vi "AlGaInPAs_prep_run_cont_dil_v11.vi"(2 "Debug Mode":bool, 3 "Elapsed Time(s)":dbl, 4 "State":enum16{"Edit", "Start", "Run", "End", "Idle"}(ring), 5 "Argument List In":string[](array[string])) -> (0 "Status Out":string, 1 "Argument List Out":string[](array[string]))   [LabVIEW 2011]
panel:
  out "GAMFC1 set val":dbl caption="R1 (0-10 sscm)" format="%.2f"
  out "Prep-In var":bool
  out "Prep-Ga var":bool
  out "Prep-Al var":bool
  out "Prep-P var":bool
  out "Prep-As var":bool
  out "prep_done":bool
  out "run started":bool
  out "first":bool=TRUE
  out "total time":dbl
  out "is OK?":bool
  out "AsH3?":bool
  out "PH3?":bool
  out "In?":bool
  out "Ga?":bool
  out "Al?":bool
  in  "Prep As":bool caption="Pre-run"
  in  "Prep P":bool caption="Pre-run"
  in  "Prep In":bool caption="Pre-run"
  in  "prep_time":dbl caption="pre-run time (s)"
  in  "Prep Al":bool caption="Pre-run"
  in  "Run As":bool caption="Run"
  in  "AsH3 Flow":dbl caption="AsH3 Flow (0-10 sccm)" format="%.2f"
  in  "P Flow":dbl caption="P Flow (0-100 sccm)" format="%.2f"
  in  "Run P":bool caption="Run"
  in  "In Flow":dbl caption="In Flow (0-100 sscm)" format="%.2f"
  in  "Run In":bool caption="Run"
  in  "Run Al":bool caption="Run"
  in  "Al Flow":dbl caption="Al Flow (0-100 sscm)" format="%.2f"
  in  "Cancel":bool
  in  "OK":bool
  out "tTotal(s) 2":dbl
  in  "Ga Tab Control":enum32{"Page 1", "Page 2"}(tab)
  in  "Ga Dilution":bool caption="Dilute"
  in  "Ga Flow":dbl caption="Ga Flow (0-10 sscm)" format="%.2f"
  in  "Run Ga":bool caption="Run"
  in  "Prep Ga":bool caption="Pre-run"
  in  "GAMFC1":dbl=1.0 caption="R1 (0-10 sscm)" format="%.2f"
  out "GAMFC2 set":dbl caption="R2 (0-100 sscm)" format="%.2f"
  in  "GAMFC3":dbl=100.0 caption="R3 (0-1000 sscm)" format="%.1f"
  out "GAMFC1 set":dbl caption="R1 (0-10 sscm)" format="%.2f"
  # "Add pre-run time to run time in editor."
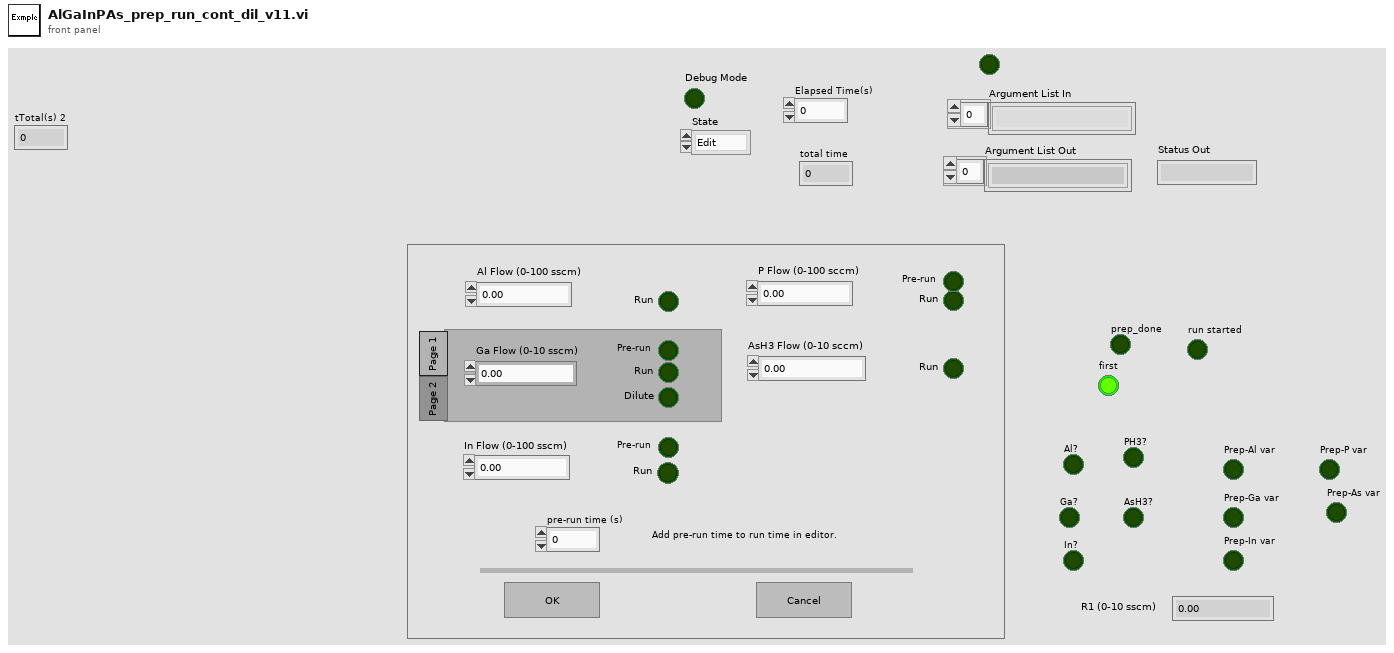
[diagram p1: front panel]
types:
  T1 = enum16{"Discrete", "Continuous", "Instantaneous", "Finite"}
  T2 = enum32{"Invalid", "Default", "Floating", "Floating/Auto-Hide", "Modal"}
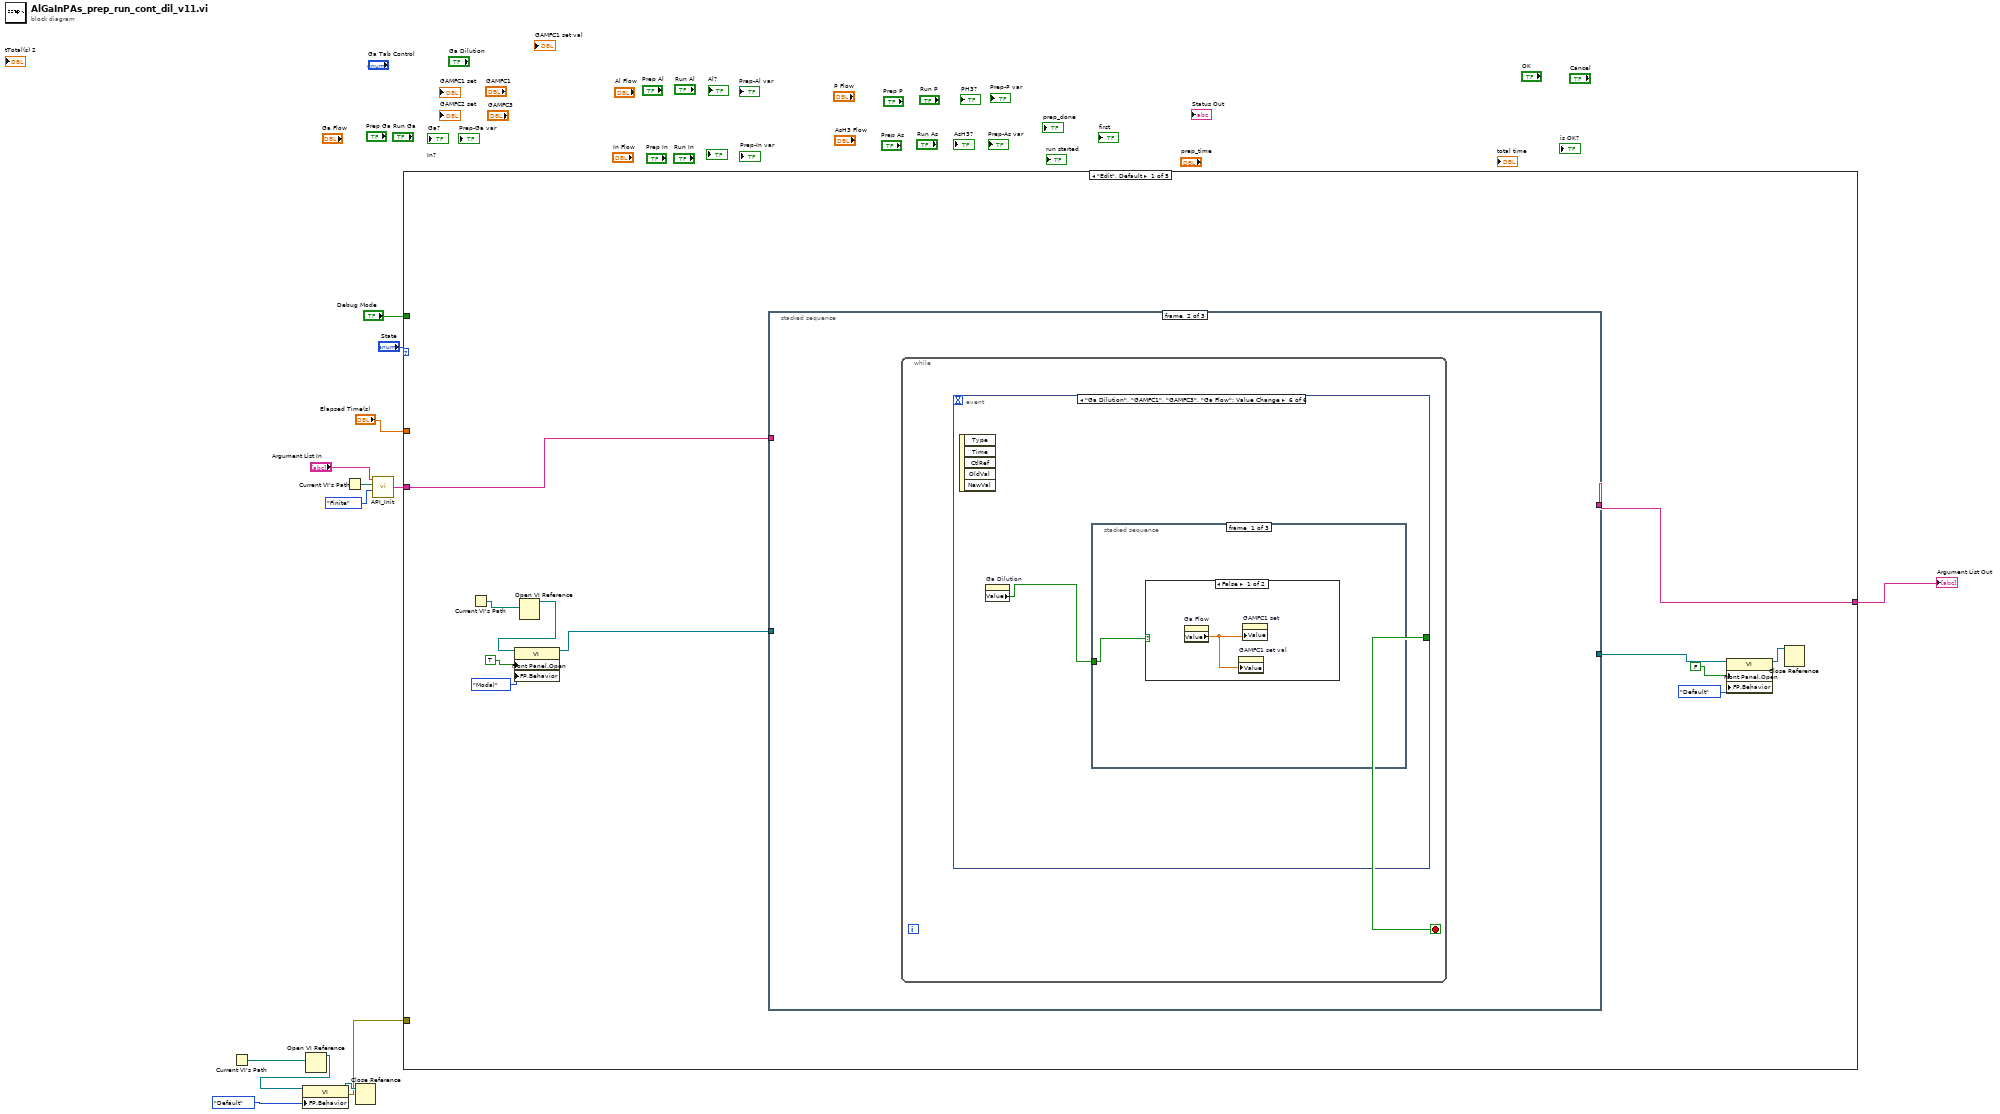
[diagram p0: block diagram]
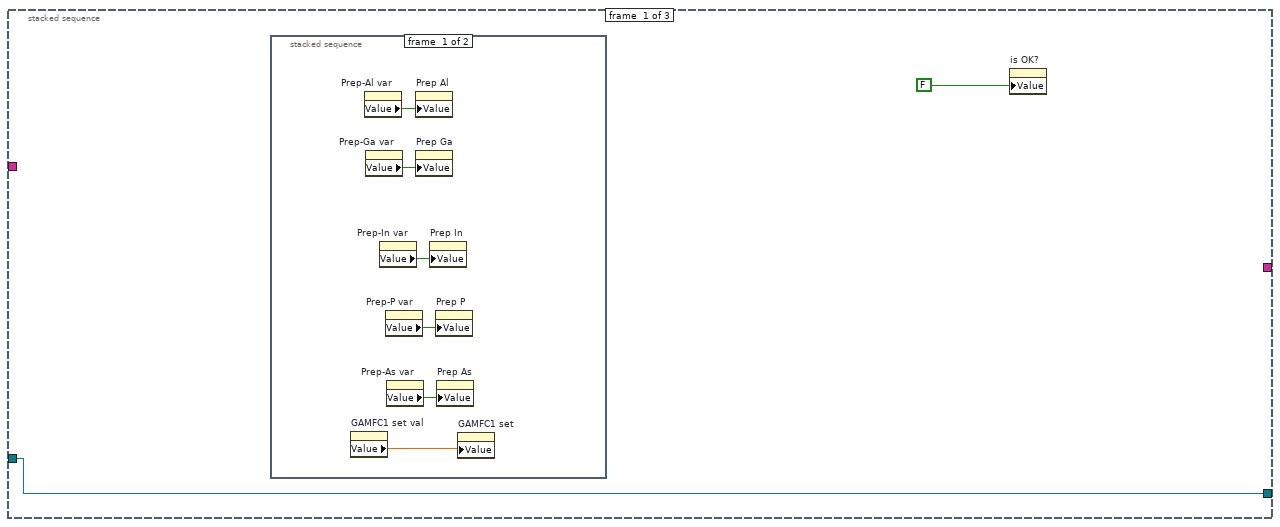
[diagram p2: hidden frame]
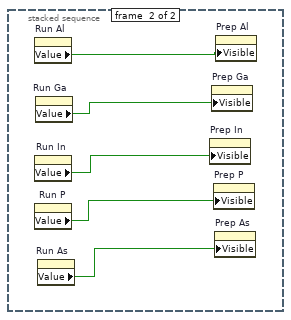
[diagram p3: hidden frame]
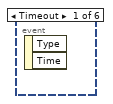
[diagram p4: hidden frame]
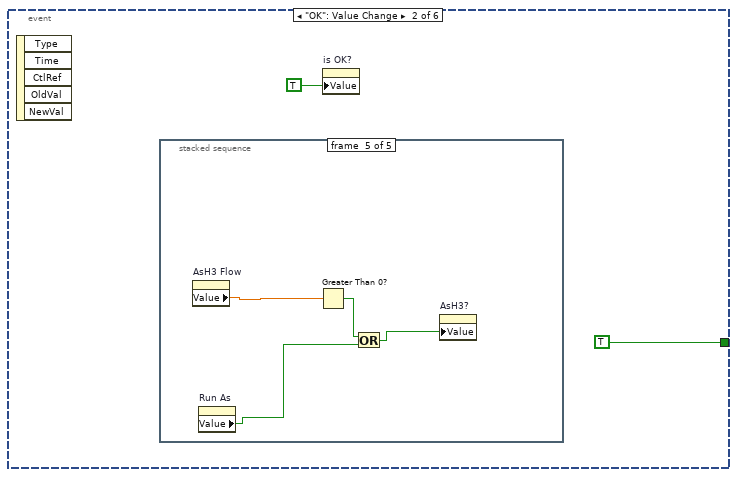
[diagram p5: hidden frame]
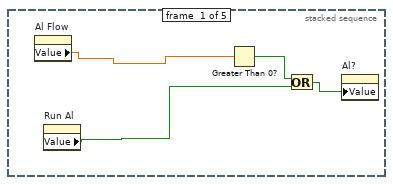
[diagram p6: hidden frame]
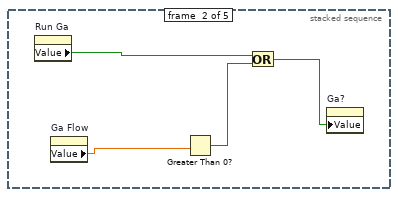
[diagram p7: hidden frame]
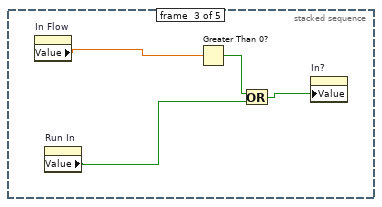
[diagram p8: hidden frame]
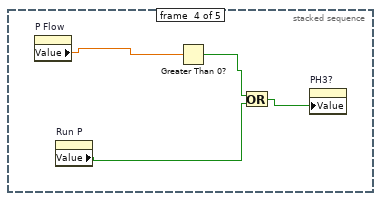
[diagram p9: hidden frame]
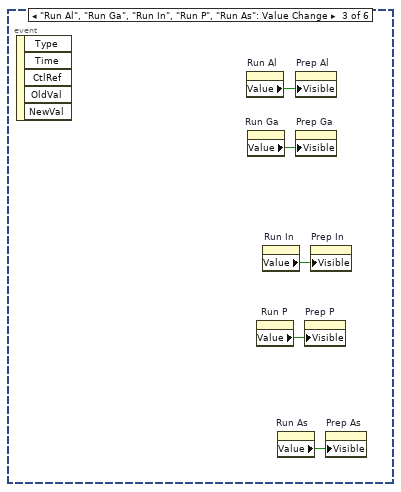
[diagram p10: hidden frame]
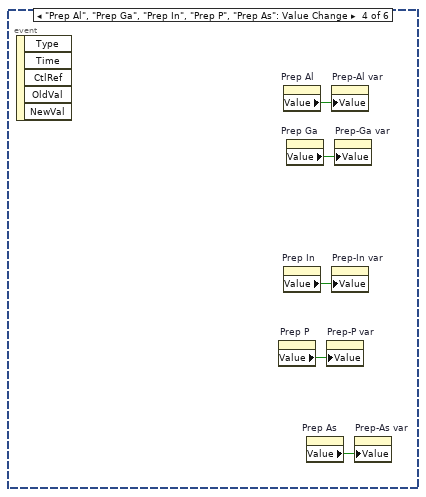
[diagram p11: hidden frame]
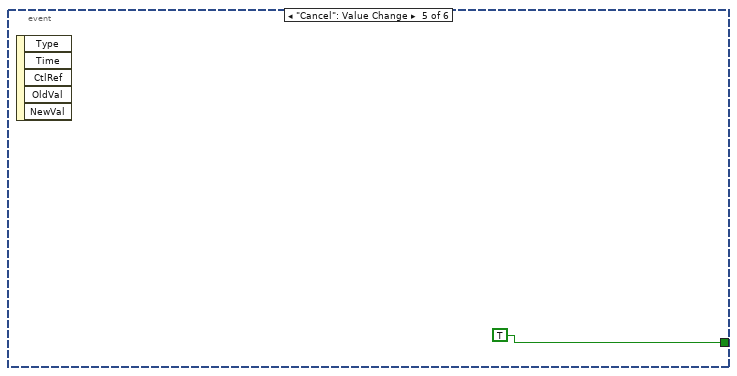
[diagram p12: hidden frame]
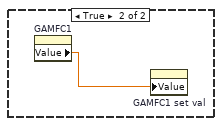
[diagram p13: hidden frame]
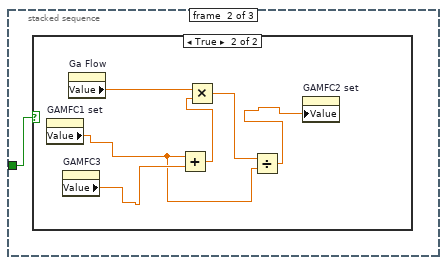
[diagram p14: hidden frame]
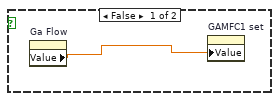
[diagram p15: hidden frame]
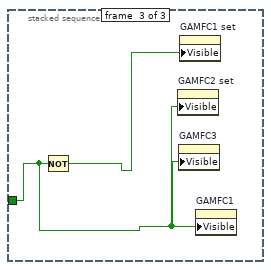
[diagram p16: hidden frame]
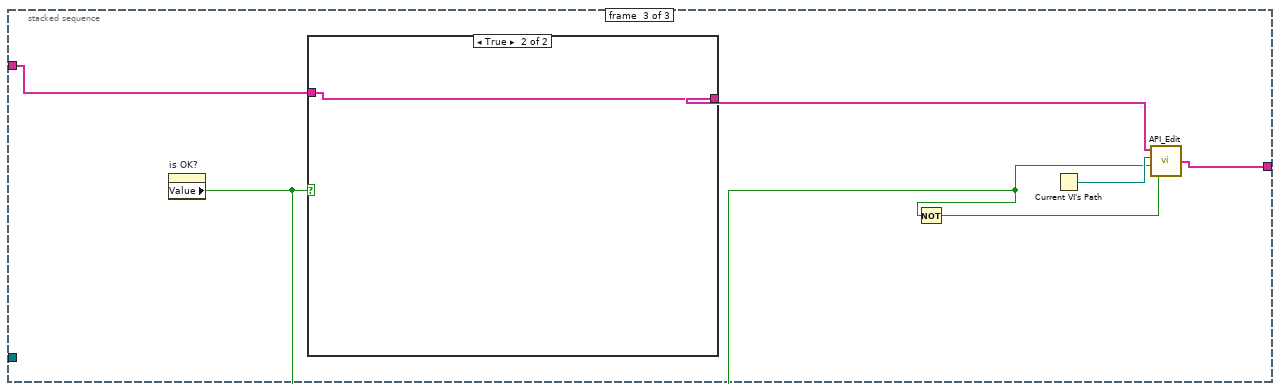
[diagram p17: hidden frame]
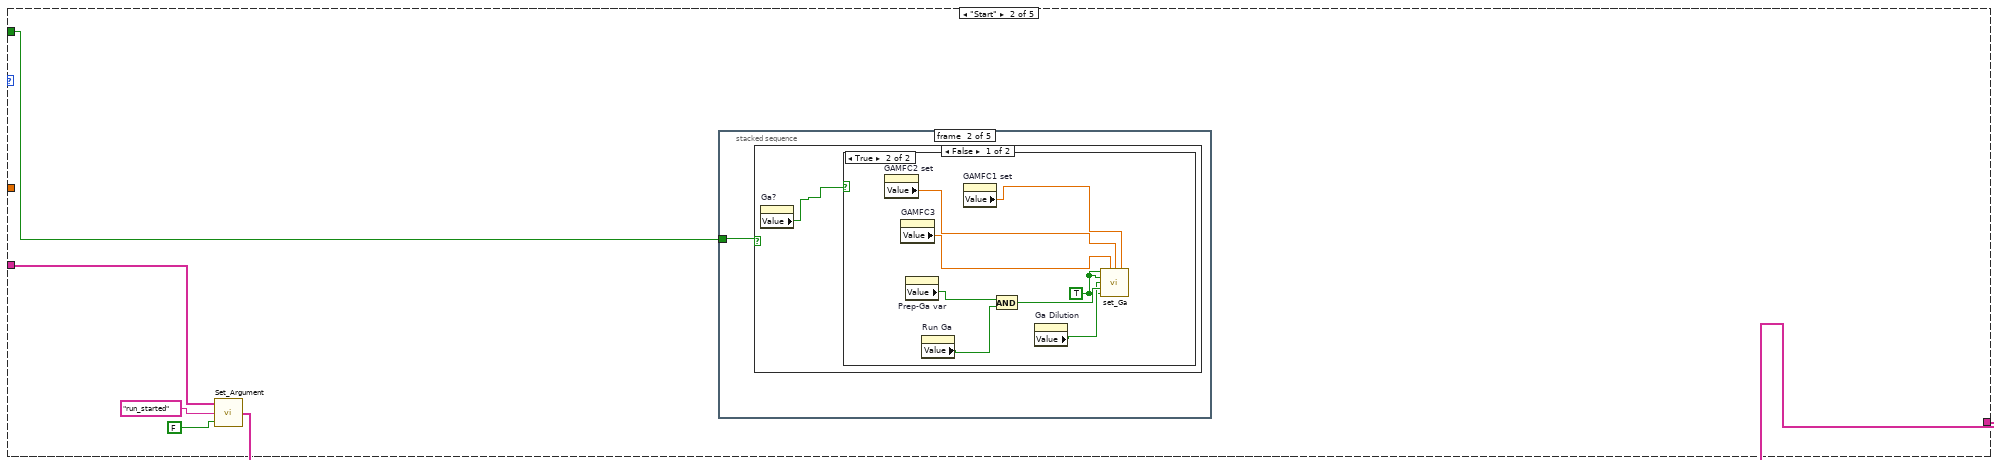
[diagram p19: hidden frame]
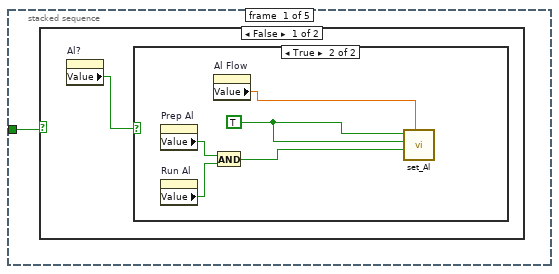
[diagram p20: hidden frame]
diagram:
  n1 = Current VI's Path() -> (path=w9:path)
  n2 = Open VI Reference(vi path=w9) -> (vi reference=w8:refnum<vi>)  [unwired: 1 in, 5 out]
  n3 = property class="VI"(reference=w8, "FP.Behavior"=T2."Default" ("Front Panel Window:Behavior")) -> (reference out=w6:refnum<vi>, error out=w5:errorcluster)  [unwired: 1 in]
  n4 = Current VI's Path() -> (path=w4:path)
  n5 = Close Reference(reference=w6) -> ()  [unwired: 1 in, 1 out]
  n6 = call "API_Init.vi"("API Mode"=T1."Finite", "VI Path"=w4, "Argument List In"="Argument List In") -> ("Argument List Out"=w1:string[])  [unwired: 1 in]
  n7 = case shown="\"Edit\", Default" "State" {
    tunnel: "Debug Mode" -> [_ w94 w148 _ _]
    tunnel: "Elapsed Time(s)" -> [_ _ w150 _ _]
    tunnel: w1 -> [w15 w96 w147 w265 w266]
    tunnel: [w14 w95 w149 w265 w266] -> w10
    tunnel: w5 -> [_ _ _ _ _]
    frame "Edit", Default {
      n8 = Current VI's Path() -> (path=w20:path)
      n9 = Open VI Reference(vi path=w20) -> (vi reference=w19:refnum<vi>)  [unwired: 1 in, 5 out]
      n10 = property class="VI"(reference=w19, "Front Panel.Open"=TRUE ("Front Panel Window:Open"), "FP.Behavior"=T2."Modal" ("Front Panel Window:Behavior")) -> (reference out=w18:refnum<vi>)  [unwired: 1 in, 1 out]
      n11 = stacked-sequence {
        tunnel: w15 -> [_ _ w89]
        tunnel: w18 -> [w26 _ _]
        tunnel: [w26 _ _] -> w22
        tunnel: [_ _ w87] -> w14
        frame #0 {
          n12 = stacked-sequence {
            frame #0 {
              n13 = property on="GAMFC1 set val" class="DigNum (strict)"() -> ("Value"=w27:dbl)  [unwired: 2 in, 2 out]
              n14 = property on="Prep-Al var" class="Bool (strict)"() -> ("Value"=w32:bool)  [unwired: 2 in, 2 out]
              n15 = property on="Prep-Ga var" class="Bool (strict)"() -> ("Value"=w31:bool)  [unwired: 2 in, 2 out]
              n16 = property on="Prep-In var" class="Bool (strict)"() -> ("Value"=w30:bool)  [unwired: 2 in, 2 out]
              n17 = property on="Prep-P var" class="Bool (strict)"() -> ("Value"=w29:bool)  [unwired: 2 in, 2 out]
              n18 = property on="Prep-As var" class="Bool (strict)"() -> ("Value"=w28:bool)  [unwired: 2 in, 2 out]
              n19 = property on="Prep Al" class="Bool (strict)"("Value"=w32) -> ()  [unwired: 2 in, 2 out]
              n20 = property on="Prep Ga" class="Bool (strict)"("Value"=w31) -> ()  [unwired: 2 in, 2 out]
              n21 = property on="Prep In" class="Bool (strict)"("Value"=w30) -> ()  [unwired: 2 in, 2 out]
              n22 = property on="Prep P" class="Bool (strict)"("Value"=w29) -> ()  [unwired: 2 in, 2 out]
              n23 = property on="Prep As" class="Bool (strict)"("Value"=w28) -> ()  [unwired: 2 in, 2 out]
              n24 = property on="GAMFC1 set" class="DigNum (strict)"("Value"=w27) -> ()  [unwired: 2 in, 2 out]
            }
            frame #1 {
              n25 = property on="Run Al" class="Bool (strict)"() -> ("Value"=w37:bool)  [unwired: 2 in, 2 out]
              n26 = property on="Run In" class="Bool (strict)"() -> ("Value"=w35:bool)  [unwired: 2 in, 2 out]
              n27 = property on="Run P" class="Bool (strict)"() -> ("Value"=w34:bool)  [unwired: 2 in, 2 out]
              n28 = property on="Run Ga" class="Bool (strict)"() -> ("Value"=w36:bool)  [unwired: 2 in, 2 out]
              n29 = property on="Run As" class="Bool (strict)"() -> ("Value"=w33:bool)  [unwired: 2 in, 2 out]
              n30 = property on="Prep In" class="Bool (strict)"("Visible"=w35) -> ()  [unwired: 2 in, 2 out]
              n31 = property on="Prep Ga" class="Bool (strict)"("Visible"=w36) -> ()  [unwired: 2 in, 2 out]
              n32 = property on="Prep P" class="Bool (strict)"("Visible"=w34) -> ()  [unwired: 2 in, 2 out]
              n33 = property on="Prep As" class="Bool (strict)"("Visible"=w33) -> ()  [unwired: 2 in, 2 out]
              n34 = property on="Prep Al" class="Bool (strict)"("Visible"=w37) -> ()  [unwired: 2 in, 2 out]
            }
          }
          n35 = property on="is OK?" class="Bool (strict)"("Value"=FALSE ("is OK?")) -> ()  [unwired: 2 in, 2 out]
        }
        frame #1 {
          n36 = while {
            stop <- w38 stop-if-true
            n37 = event shown="[5] \"Ga Dilution\", \"GAMFC1\", \"GAMFC3\", \"Ga Flow\": Value Change" {
              selector: _ -> [_ _ _ _ _ _]
              dyn-events: _ -> [_ _ _ _ _ _]
              timeout: _ -> [_ _ _ _ _ _]
              tunnel: [_ TRUE _ _ TRUE _] -> w38
              event Timeout {
                n38 = event-data() -> ()  [unwired: 1 in, 2 out]
              }
              event "OK": Value Change {
                n39 = event-data() -> ()  [unwired: 1 in, 5 out]
                n40 = stacked-sequence {
                  frame #0 {
                    n41 = property on="Al Flow" class="DigNum (strict)"() -> ("Value"=w43:dbl)  [unwired: 2 in, 2 out]
                    n42 = property on="Run Al" class="Bool (strict)"() -> ("Value"=w42:bool)  [unwired: 2 in, 2 out]
                    n43 = Greater Than 0?(x=w43) -> (x > 0?=w44:bool)
                    n44 = Or(x=w44, y=w42) -> (x .or. y?=w41:bool)
                    n45 = property on="Al?" class="Bool (strict)"("Value"=w41) -> ()  [unwired: 2 in, 2 out]
                  }
                  frame #1 {
                    n46 = property on="Run Ga" class="Bool (strict)"() -> ("Value"=w46:bool)  [unwired: 2 in, 2 out]
                    n47 = property on="Ga Flow" class="DigNum (strict)"() -> ("Value"=w47:dbl)  [unwired: 2 in, 2 out]
                    n48 = Greater Than 0?(x=w47) -> (x > 0?=w48:bool)
                    n49 = Or(x=w46, y=w48) -> (x .or. y?=w45:bool)
                    n50 = property on="Ga?" class="Bool (strict)"("Value"=w45) -> ()  [unwired: 2 in, 2 out]
                  }
                  frame #2 {
                    n51 = property on="In Flow" class="DigNum (strict)"() -> ("Value"=w50:dbl)  [unwired: 2 in, 2 out]
                    n52 = property on="Run In" class="Bool (strict)"() -> ("Value"=w51:bool)  [unwired: 2 in, 2 out]
                    n53 = Greater Than 0?(x=w50) -> (x > 0?=w52:bool)
                    n54 = Or(x=w52, y=w51) -> (x .or. y?=w49:bool)
                    n55 = property on="In?" class="Bool (strict)"("Value"=w49) -> ()  [unwired: 2 in, 2 out]
                  }
                  frame #3 {
                    n56 = property on="P Flow" class="DigNum (strict)"() -> ("Value"=w55:dbl)  [unwired: 2 in, 2 out]
                    n57 = property on="Run P" class="Bool (strict)"() -> ("Value"=w54:bool)  [unwired: 2 in, 2 out]
                    n58 = Greater Than 0?(x=w55) -> (x > 0?=w56:bool)
                    n59 = Or(x=w56, y=w54) -> (x .or. y?=w53:bool)
                    n60 = property on="PH3?" class="Bool (strict)"("Value"=w53) -> ()  [unwired: 2 in, 2 out]
                  }
                  frame #4 {
                    n61 = property on="AsH3 Flow" class="DigNum (strict)"() -> ("Value"=w59:dbl)  [unwired: 2 in, 2 out]
                    n62 = property on="Run As" class="Bool (strict)"() -> ("Value"=w58:bool)  [unwired: 2 in, 2 out]
                    n63 = Greater Than 0?(x=w59) -> (x > 0?=w60:bool)
                    n64 = Or(x=w60, y=w58) -> (x .or. y?=w57:bool)
                    n65 = property on="AsH3?" class="Bool (strict)"("Value"=w57) -> ()  [unwired: 2 in, 2 out]
                  }
                }
                n66 = property on="is OK?" class="Bool (strict)"("Value"=TRUE ("is OK?")) -> ()  [unwired: 2 in, 2 out]
              }
              event "Run Al", "Run Ga", "Run In", "Run P", "Run As": Value Change {
                n67 = event-data() -> ()  [unwired: 1 in, 5 out]
                n68 = property on="Run Al" class="Bool (strict)"() -> ("Value"=w65:bool)  [unwired: 2 in, 2 out]
                n69 = property on="Run Ga" class="Bool (strict)"() -> ("Value"=w64:bool)  [unwired: 2 in, 2 out]
                n70 = property on="Run P" class="Bool (strict)"() -> ("Value"=w61:bool)  [unwired: 2 in, 2 out]
                n71 = property on="Run In" class="Bool (strict)"() -> ("Value"=w63:bool)  [unwired: 2 in, 2 out]
                n72 = property on="Run As" class="Bool (strict)"() -> ("Value"=w62:bool)  [unwired: 2 in, 2 out]
                n73 = property on="Prep Al" class="Bool (strict)"("Visible"=w65) -> ()  [unwired: 2 in, 2 out]
                n74 = property on="Prep Ga" class="Bool (strict)"("Visible"=w64) -> ()  [unwired: 2 in, 2 out]
                n75 = property on="Prep P" class="Bool (strict)"("Visible"=w61) -> ()  [unwired: 2 in, 2 out]
                n76 = property on="Prep In" class="Bool (strict)"("Visible"=w63) -> ()  [unwired: 2 in, 2 out]
                n77 = property on="Prep As" class="Bool (strict)"("Visible"=w62) -> ()  [unwired: 2 in, 2 out]
              }
              event "Prep Al", "Prep Ga", "Prep In", "Prep P", "Prep As": Value Change {
                n78 = event-data() -> ()  [unwired: 1 in, 5 out]
                n79 = property on="Prep P" class="Bool (strict)"() -> ("Value"=w67:bool)  [unwired: 2 in, 2 out]
                n80 = property on="Prep Al" class="Bool (strict)"() -> ("Value"=w70:bool)  [unwired: 2 in, 2 out]
                n81 = property on="Prep In" class="Bool (strict)"() -> ("Value"=w68:bool)  [unwired: 2 in, 2 out]
                n82 = property on="Prep Ga" class="Bool (strict)"() -> ("Value"=w69:bool)  [unwired: 2 in, 2 out]
                n83 = property on="Prep As" class="Bool (strict)"() -> ("Value"=w66:bool)  [unwired: 2 in, 2 out]
                n84 = property on="Prep-P var" class="Bool (strict)"("Value"=w67) -> ()  [unwired: 2 in, 2 out]
                n85 = property on="Prep-Al var" class="Bool (strict)"("Value"=w70) -> ()  [unwired: 2 in, 2 out]
                n86 = property on="Prep-In var" class="Bool (strict)"("Value"=w68) -> ()  [unwired: 2 in, 2 out]
                n87 = property on="Prep-Ga var" class="Bool (strict)"("Value"=w69) -> ()  [unwired: 2 in, 2 out]
                n88 = property on="Prep-As var" class="Bool (strict)"("Value"=w66) -> ()  [unwired: 2 in, 2 out]
              }
              event "Cancel": Value Change {
                n89 = event-data() -> ()  [unwired: 1 in, 5 out]
              }
              event "Ga Dilution", "GAMFC1", "GAMFC3", "Ga Flow": Value Change {
                n90 = event-data() -> ()  [unwired: 1 in, 5 out]
                n91 = property on="Ga Dilution" class="Bool (strict)"() -> ("Value"=w72:bool)  [unwired: 2 in, 2 out]
                n92 = stacked-sequence {
                  tunnel: w72 -> [w73 w76 w84]
                  frame #0 {
                    n93 = case shown="False" w73 {
                      frame False {
                        n94 = property on="Ga Flow" class="DigNum (strict)"() -> ("Value"=w74:dbl)  [unwired: 2 in, 2 out]
                        n95 = property on="GAMFC1 set val" class="DigNum (strict)"("Value"=w74) -> ()  [unwired: 2 in, 2 out]
                        n96 = property on="GAMFC1 set" class="DigNum (strict)"("Value"=w74) -> ()  [unwired: 2 in, 2 out]
                      }
                      frame True {
                        n97 = property on="GAMFC1" class="DigNum (strict)"() -> ("Value"=w75:dbl)  [unwired: 2 in, 2 out]
                        n98 = property on="GAMFC1 set val" class="DigNum (strict)"("Value"=w75) -> ()  [unwired: 2 in, 2 out]
                      }
                    }
                  }
                  frame #1 {
                    n99 = case shown="True" w76 {
                      frame False {
                        n100 = property on="Ga Flow" class="DigNum (strict)"() -> ("Value"=w77:dbl)  [unwired: 2 in, 2 out]
                        n101 = property on="GAMFC1 set" class="DigNum (strict)"("Value"=w77) -> ()  [unwired: 2 in, 2 out]
                      }
                      frame True {
                        n102 = property on="GAMFC1 set" class="DigNum (strict)"() -> ("Value"=w78:dbl)  [unwired: 2 in, 2 out]
                        n103 = property on="GAMFC3" class="DigNum (strict)"() -> ("Value"=w80:dbl)  [unwired: 2 in, 2 out]
                        n104 = property on="Ga Flow" class="DigNum (strict)"() -> ("Value"=w81:dbl)  [unwired: 2 in, 2 out]
                        n105 = Add(x=w78, y=w80) -> (x+y=w83:dbl)
                        n106 = Multiply(x=w81, y=w83) -> (x*y=w79:dbl)
                        n107 = Divide(x=w79, y=w78) -> (x/y=w82:dbl)
                        n108 = property on="GAMFC2 set" class="DigNum (strict)"("Value"=w82) -> ()  [unwired: 2 in, 2 out]
                      }
                    }
                  }
                  frame #2 {
                    n109 = Not(x=w84) -> (.not. x?=w85:bool)
                    n110 = property on="GAMFC2 set" class="DigNum (strict)"("Visible"=w84) -> ()  [unwired: 2 in, 2 out]
                    n111 = property on="GAMFC3" class="DigNum (strict)"("Visible"=w84) -> ()  [unwired: 2 in, 2 out]
                    n112 = property on="GAMFC1 set" class="DigNum (strict)"("Visible"=w85) -> ()  [unwired: 2 in, 2 out]
                    n113 = property on="GAMFC1" class="DigNum (strict)"("Visible"=w84) -> ()  [unwired: 2 in, 2 out]
                  }
                }
              }
            }
          }
        }
        frame #2 {
          n114 = property on="is OK?" class="Bool (strict)"() -> ("Value"=w86:bool)  [unwired: 2 in, 2 out]
          n115 = case shown="True" w86 {
            tunnel: w89 -> [w92 w93]
            tunnel: [w92 w93] -> w88
            frame False {
            }
            frame True {
            }
          }
          n116 = Not(x=w86) -> (.not. x?=w91:bool)
          n117 = Current VI's Path() -> (path=w90:path)
          n118 = call "API_Edit.vi"("Cancel"=w91, "OK"=w86, "VI Path"=w90, "Argument List In"=w88) -> ("Argument List Out"=w87:string[])
        }
      }
      n119 = property class="VI"(reference=w22, "Front Panel.Open"=FALSE ("Front Panel Window:Open"), "FP.Behavior"=T2."Default" ("Front Panel Window:Behavior")) -> (reference out=w23:refnum<vi>)  [unwired: 1 in, 1 out]
      n120 = Close Reference(reference=w23) -> ()  [unwired: 1 in, 1 out]
    }
    frame "Start" {
      n121 = call "Set_Argument.vi"("Enable"=FALSE, "Argument"="run_started", "Argument List In"=w96) -> ("Argument List Out"=w95:string[])
      n122 = stacked-sequence {
        tunnel: w94 -> [w99 w108 w120 w129 w138]
        frame #0 {
          n123 = case shown="False" w99 {
            frame False {
              n124 = property on="Al?" class="Bool (strict)"() -> ("Value"=w100:bool)  [unwired: 2 in, 2 out]
              n125 = case shown="True" w100 {
                frame False {
                  w101 = FALSE ("Al Active")
                  n126 = call "set_Al.vi"("Aluminum Flow"=0.0, "Al Remote"=w101, "Al Run"=w101, "Al Bubbler"=w101, "Al Active"=w101) -> ()  [unwired: 5 out]
                }
                frame True {
                  w107 = TRUE ("Al Active")
                  n127 = property on="Prep Al" class="Bool (strict)"() -> ("Value"=w105:bool)  [unwired: 2 in, 2 out]
                  n128 = property on="Run Al" class="Bool (strict)"() -> ("Value"=w104:bool)  [unwired: 2 in, 2 out]
                  n129 = property on="Al Flow" class="DigNum (strict)"() -> ("Value"=w106:dbl)  [unwired: 2 in, 2 out]
                  n130 = And(x=w105, y=w104) -> (x .and. y?=w103:bool)
                  n131 = call "set_Al.vi"("Aluminum Flow"=w106, "Al Run"=w103, "Al Bubbler"=w107, "Al Active"=w107) -> ()  [unwired: 1 in, 5 out]
                }
              }
            }
            frame True {
            }
          }
        }
        frame #1 {
          n132 = case shown="False" w108 {
            frame False {
              n133 = property on="Ga?" class="Bool (strict)"() -> ("Value"=w109:bool)  [unwired: 2 in, 2 out]
              n134 = case shown="True" w109 {
                frame False {
                  w111 = FALSE ("Ga Active")
                  w110 = 0.0 ("Ga Flow 1")
                  n135 = call "set_Ga.vi"("Ga Active"=w111, "Ga Flow 3"=w110, "Ga Flow 2"=w110, "Ga Flow 1"=w110, "Ga Bubbler"=w111, "Ga H2 Dilute"=w111, "Ga Run"=w111, "Ga Remote"=w111) -> ()  [unwired: 8 out]
                }
                frame True {
                  w112 = TRUE ("Ga Active")
                  n136 = property on="GAMFC2 set" class="DigNum (strict)"() -> ("Value"=w114:dbl)  [unwired: 2 in, 2 out]
                  n137 = property on="GAMFC3" class="DigNum (strict)"() -> ("Value"=w113:dbl)  [unwired: 2 in, 2 out]
                  n138 = property on="Prep-Ga var" class="Bool (strict)"() -> ("Value"=w116:bool)  [unwired: 2 in, 2 out]
                  n139 = property on="Run Ga" class="Bool (strict)"() -> ("Value"=w117:bool)  [unwired: 2 in, 2 out]
                  n140 = property on="GAMFC1 set" class="DigNum (strict)"() -> ("Value"=w115:dbl)  [unwired: 2 in, 2 out]
                  n141 = And(x=w116, y=w117) -> (x .and. y?=w119:bool)
                  n142 = property on="Ga Dilution" class="Bool (strict)"() -> ("Value"=w118:bool)  [unwired: 2 in, 2 out]
                  n143 = call "set_Ga.vi"("Ga Active"=w112, "Ga Flow 3"=w113, "Ga Flow 2"=w114, "Ga Flow 1"=w115, "Ga Bubbler"=w112, "Ga H2 Dilute"=w118, "Ga Run"=w119, "Ga Remote"=w112) -> ()  [unwired: 8 in]
                }
              }
            }
            frame True {
            }
          }
        }
        frame #2 {
          n144 = case shown="False" w120 {
            frame False {
              n145 = property on="In?" class="Bool (strict)"() -> ("Value"=w121:bool)  [unwired: 2 in, 2 out]
              n146 = case shown="True" w121 {
                frame False {
                  w123 = FALSE ("In Remote")
                  n147 = call "set_In.vi"("Indium Flow"=0.0, "In Remote"=w123, "In Run"=w123, "In Bubbler"=w123, "In Active"=w123) -> ()  [unwired: 5 out]
                }
                frame True {
                  w128 = TRUE ("In Run")
                  n148 = property on="Run In" class="Bool (strict)"() -> ("Value"=w125:bool)  [unwired: 2 in, 2 out]
                  n149 = property on="Prep In" class="Bool (strict)"() -> ("Value"=w126:bool)  [unwired: 2 in, 2 out]
                  n150 = And(x=w126, y=w125) -> (x .and. y?=w124:bool)
                  n151 = property on="In Flow" class="DigNum (strict)"() -> ("Value"=w127:dbl)  [unwired: 2 in, 2 out]
                  n152 = call "set_In.vi"("Indium Flow"=w127, "In Run"=w124, "In Bubbler"=w128, "In Active"=w128) -> ()  [unwired: 1 in, 5 out]
                }
              }
            }
            frame True {
            }
          }
        }
        frame #3 {
          n153 = case shown="False" w129 {
            frame False {
              n154 = property on="PH3?" class="Bool (strict)"() -> ("Value"=w130:bool)  [unwired: 2 in, 2 out]
              n155 = case shown="True" w130 {
                frame False {
                  w131 = FALSE ("P_Gas Active")
                  n156 = call "set_P_gas.vi"("P_Gas Active"=w131, "P_Gas Flow"=0.0, "P_Gas In"=w131, "P_Gas H2 In"=w131, "P_Gas Run"=w131, "P_Gas Remote"=w131) -> ()  [unwired: 10 out]
                }
                frame True {
                  w137 = TRUE ("P_Gas Active")
                  n157 = property on="P Flow" class="DigNum (strict)"() -> ("Value"=w136:dbl)  [unwired: 2 in, 2 out]
                  n158 = property on="Prep P" class="Bool (strict)"() -> ("Value"=w135:bool)  [unwired: 2 in, 2 out]
                  n159 = property on="Run P" class="Bool (strict)"() -> ("Value"=w134:bool)  [unwired: 2 in, 2 out]
                  n160 = And(x=w135, y=w134) -> (x .and. y?=w133:bool)
                  n161 = call "set_P_gas.vi"("P_Gas Active"=w137, "P_Gas Flow"=w136, "P_Gas In"=w137, "P_Gas Run"=w133) -> ()  [unwired: 2 in, 10 out]
                }
              }
            }
            frame True {
            }
          }
        }
        frame #4 {
          n162 = case shown="False" w138 {
            frame False {
              n163 = property on="AsH3?" class="Bool (strict)"() -> ("Value"=w139:bool)  [unwired: 2 in, 2 out]
              n164 = case shown="True" w139 {
                frame False {
                  w140 = FALSE ("As_Gas Active")
                  n165 = call "set_As_gas.vi"("As_Gas Active"=w140, "As_Gas Flow"=0.0, "As_Gas In"=w140, "As_Gas H2"=w140, "As_Gas Run"=w140, "As_Gas Remote"=w140) -> ()  [unwired: 10 in]
                }
                frame True {
                  w146 = TRUE ("As_Gas Active")
                  n166 = property on="Prep As" class="Bool (strict)"() -> ("Value"=w143:bool)  [unwired: 2 in, 2 out]
                  n167 = property on="Run As" class="Bool (strict)"() -> ("Value"=w144:bool)  [unwired: 2 in, 2 out]
                  n168 = property on="AsH3 Flow" class="DigNum (strict)"() -> ("Value"=w145:dbl)  [unwired: 2 in, 2 out]
                  n169 = And(x=w143, y=w144) -> (x .and. y?=w142:bool)
                  n170 = call "set_As_gas.vi"("As_Gas Active"=w146, "As_Gas Flow"=w145, "As_Gas In"=w146, "As_Gas Run"=w142) -> ()  [unwired: 12 in]
                }
              }
            }
            frame True {
            }
          }
        }
      }
    }
    frame "Run" {
      n171 = stacked-sequence {
        tunnel: w150 -> [_ w155 _ _]
        tunnel: w147 -> [w152 _ _ w209]
        tunnel: [_ _ _ w208] -> w149
        tunnel: w148 -> [_ _ _ w210]
        frame #0 {
          n172 = call "Get_Argument.vi"("Argument"="run_started", "Argument List"=w152) -> ("Enabled"=w151:bool)
          n173 = local write "run started"(w151) -> ()
        }
        frame #1 {
          n174 = property on="prep_time" class="DigNum (strict)"() -> ("Value"=w156:dbl)  [unwired: 2 in, 2 out]
          n175 = Greater Or Equal?(x=w155, y=w156) -> (x >= y?=w154:bool)
          n176 = local write "prep_done"(w154) -> ()
        }
        frame #2 {
          n177 = local read "run started"() -> (w158:bool)
          n178 = Not(x=w158) -> (.not. x?=w157:bool)
          n179 = stacked-sequence {
            tunnel: w157 -> [w160 w164 w173 w182 w191 w200]
            frame #0 {
              n180 = case shown="True" w160 {
                tunnel: ["run: " "pre-run: "] -> w159
                frame False {
                }
                frame True {
                }
              }
              n181 = property on="Status Out" class="Str"("Value"=w159) -> ()  [unwired: 2 in, 2 out]
            }
            frame #1 {
              n182 = property on="Status Out" class="Str"() -> ("Value"=w170:string)  [unwired: 2 in, 2 out]
              n183 = property on="Al?" class="Bool (strict)"() -> ("Value"=w171:bool)  [unwired: 2 in, 2 out]
              n184 = property on="Run Al" class="Bool (strict)"() -> ("Value"=w163:bool)  [unwired: 2 in, 2 out]
              n185 = property on="Prep Al" class="Bool (strict)"() -> ("Value"=w165:bool)  [unwired: 2 in, 2 out]
              n186 = call "flow_strings.vi"("string in"=w170, "is first in?"=TRUE, "use source?"=w171, "name"="Al", "run source?"=w163, "prep source?"=w165, "is prep?"=w164) -> ("string out"=w169:string, "is first out?"=w168:bool)
              n187 = property on="Status Out" class="Str"("Value"=w169) -> ()  [unwired: 2 in, 2 out]
              n188 = property on="first" class="Bool (strict)"("Value"=w168) -> ()  [unwired: 2 in, 2 out]
            }
            frame #2 {
              n189 = property on="first" class="Bool (strict)"() -> ("Value"=w176:bool)  [unwired: 2 in, 2 out]
              n190 = property on="Status Out" class="Str"() -> ("Value"=w179:string)  [unwired: 2 in, 2 out]
              n191 = property on="Ga?" class="Bool (strict)"() -> ("Value"=w177:bool)  [unwired: 2 in, 2 out]
              n192 = property on="Run Ga" class="Bool (strict)"() -> ("Value"=w172:bool)  [unwired: 2 in, 2 out]
              n193 = property on="Prep Ga" class="Bool (strict)"() -> ("Value"=w174:bool)  [unwired: 2 in, 2 out]
              n194 = call "flow_strings.vi"("string in"=w179, "is first in?"=w176, "use source?"=w177, "name"="Ga", "run source?"=w172, "prep source?"=w174, "is prep?"=w173) -> ("string out"=w180:string, "is first out?"=w175:bool)
              n195 = property on="Status Out" class="Str"("Value"=w180) -> ()  [unwired: 2 in, 2 out]
              n196 = property on="first" class="Bool (strict)"("Value"=w175) -> ()  [unwired: 2 in, 2 out]
            }
            frame #3 {
              n197 = property on="first" class="Bool (strict)"() -> ("Value"=w186:bool)  [unwired: 2 in, 2 out]
              n198 = property on="Status Out" class="Str"() -> ("Value"=w188:string)  [unwired: 2 in, 2 out]
              n199 = property on="In?" class="Bool (strict)"() -> ("Value"=w189:bool)  [unwired: 2 in, 2 out]
              n200 = property on="Run In" class="Bool (strict)"() -> ("Value"=w181:bool)  [unwired: 2 in, 2 out]
              n201 = property on="Prep In" class="Bool (strict)"() -> ("Value"=w183:bool)  [unwired: 2 in, 2 out]
              n202 = call "flow_strings.vi"("string in"=w188, "is first in?"=w186, "use source?"=w189, "name"="In", "run source?"=w181, "prep source?"=w183, "is prep?"=w182) -> ("string out"=w185:string, "is first out?"=w184:bool)
              n203 = property on="Status Out" class="Str"("Value"=w185) -> ()  [unwired: 2 in, 2 out]
              n204 = property on="first" class="Bool (strict)"("Value"=w184) -> ()  [unwired: 2 in, 2 out]
            }
            frame #4 {
              n205 = property on="first" class="Bool (strict)"() -> ("Value"=w194:bool)  [unwired: 2 in, 2 out]
              n206 = property on="Status Out" class="Str"() -> ("Value"=w196:string)  [unwired: 2 in, 2 out]
              n207 = property on="PH3?" class="Bool (strict)"() -> ("Value"=w197:bool)  [unwired: 2 in, 2 out]
              n208 = property on="Run P" class="Bool (strict)"() -> ("Value"=w190:bool)  [unwired: 2 in, 2 out]
              n209 = property on="Prep P" class="Bool (strict)"() -> ("Value"=w192:bool)  [unwired: 2 in, 2 out]
              n210 = call "flow_strings.vi"("string in"=w196, "is first in?"=w194, "use source?"=w197, "name"="P", "run source?"=w190, "prep source?"=w192, "is prep?"=w191) -> ("string out"=w195:string, "is first out?"=w193:bool)
              n211 = property on="Status Out" class="Str"("Value"=w195) -> ()  [unwired: 2 in, 2 out]
              n212 = property on="first" class="Bool (strict)"("Value"=w193) -> ()  [unwired: 2 in, 2 out]
            }
            frame #5 {
              n213 = property on="first" class="Bool (strict)"() -> ("Value"=w203:bool)  [unwired: 2 in, 2 out]
              n214 = property on="Status Out" class="Str"() -> ("Value"=w205:string)  [unwired: 2 in, 2 out]
              n215 = property on="AsH3?" class="Bool (strict)"() -> ("Value"=w206:bool)  [unwired: 2 in, 2 out]
              n216 = property on="Run As" class="Bool (strict)"() -> ("Value"=w199:bool)  [unwired: 2 in, 2 out]
              n217 = property on="Prep As" class="Bool (strict)"() -> ("Value"=w201:bool)  [unwired: 2 in, 2 out]
              n218 = call "flow_strings.vi"("string in"=w205, "is first in?"=w203, "use source?"=w206, "name"="As", "run source?"=w199, "prep source?"=w201, "is prep?"=w200) -> ("string out"=w202:string, "is first out?"=w204:bool)
              n219 = property on="Status Out" class="Str"("Value"=w202) -> ()  [unwired: 2 in, 2 out]
              n220 = property on="first" class="Bool (strict)"("Value"=w204) -> ()  [unwired: 2 in, 2 out]
            }
          }
        }
        frame #3 {
          n221 = local read "run started"() -> (w213:bool)
          n222 = local read "prep_done"() -> (w211:bool)
          n223 = Not(x=w213) -> (.not. x?=w214:bool)
          n224 = And(x=w211, y=w214) -> (x .and. y?=w212:bool)
          n225 = stacked-sequence {
            tunnel: w212 -> [w218]
            tunnel: w210 -> [w217]
            tunnel: w209 -> [w216]
            tunnel: [w215] -> w208
            frame #0 {
              n226 = case shown="True" w218 {
                tunnel: w217 -> [_ w222]
                tunnel: w216 -> [w219 w221]
                tunnel: [w219 w220] -> w215
                frame False {
                }
                frame True {
                  n227 = stacked-sequence {
                    tunnel: w222 -> [w223 w230 w240 w247 w254 _]
                    tunnel: w221 -> [_ _ _ _ _ w262]
                    tunnel: [_ _ _ _ _ w261] -> w220
                    frame #0 {
                      n228 = case shown="False" w223 {
                        frame False {
                          n229 = property on="Al?" class="Bool (strict)"() -> ("Value"=w224:bool)  [unwired: 2 in, 2 out]
                          n230 = case shown="True" w224 {
                            frame False {
                              w225 = FALSE ("Al Active")
                              n231 = call "set_Al.vi"("Aluminum Flow"=0.0, "Al Remote"=w225, "Al Run"=w225, "Al Bubbler"=w225, "Al Active"=w225) -> ()  [unwired: 5 out]
                            }
                            frame True {
                              w229 = TRUE ("Al Active")
                              n232 = property on="Al Flow" class="DigNum (strict)"() -> ("Value"=w228:dbl)  [unwired: 2 in, 2 out]
                              n233 = property on="Run Al" class="Bool (strict)"() -> ("Value"=w227:bool)  [unwired: 2 in, 2 out]
                              n234 = call "set_Al.vi"("Aluminum Flow"=w228, "Al Run"=w227, "Al Bubbler"=w229, "Al Active"=w229) -> ()  [unwired: 1 in, 5 out]
                            }
                          }
                        }
                        frame True {
                        }
                      }
                    }
                    frame #1 {
                      n235 = case shown="False" w230 {
                        frame False {
                          n236 = property on="Ga?" class="Bool (strict)"() -> ("Value"=w231:bool)  [unwired: 2 in, 2 out]
                          n237 = case shown="True" w231 {
                            frame False {
                              w233 = FALSE ("Ga Active")
                              w232 = 0.0 ("Ga Flow 1")
                              n238 = call "set_Ga.vi"("Ga Active"=w233, "Ga Flow 3"=w232, "Ga Flow 2"=w232, "Ga Flow 1"=w232, "Ga Bubbler"=w233, "Ga H2 Dilute"=w233, "Ga Run"=w233, "Ga Remote"=w233) -> ()  [unwired: 8 out]
                            }
                            frame True {
                              w234 = TRUE ("Ga Active")
                              n239 = property on="Ga Dilution" class="Bool (strict)"() -> ("Value"=w235:bool)  [unwired: 2 in, 2 out]
                              n240 = property on="Run Ga" class="Bool (strict)"() -> ("Value"=w236:bool)  [unwired: 2 in, 2 out]
                              n241 = property on="GAMFC3" class="DigNum (strict)"() -> ("Value"=w237:dbl)  [unwired: 2 in, 2 out]
                              n242 = property on="GAMFC2 set" class="DigNum (strict)"() -> ("Value"=w238:dbl)  [unwired: 2 in, 2 out]
                              n243 = property on="GAMFC1 set" class="DigNum (strict)"() -> ("Value"=w239:dbl)  [unwired: 2 in, 2 out]
                              n244 = call "set_Ga.vi"("Ga Active"=w234, "Ga Flow 3"=w237, "Ga Flow 2"=w238, "Ga Flow 1"=w239, "Ga Bubbler"=w234, "Ga H2 Dilute"=w235, "Ga Run"=w236, "Ga Remote"=w234) -> ()  [unwired: 8 in]
                            }
                          }
                        }
                        frame True {
                        }
                      }
                    }
                    frame #2 {
                      n245 = case shown="False" w240 {
                        frame False {
                          n246 = property on="In?" class="Bool (strict)"() -> ("Value"=w241:bool)  [unwired: 2 in, 2 out]
                          n247 = case shown="True" w241 {
                            frame False {
                              w243 = FALSE ("In Remote")
                              n248 = call "set_In.vi"("Indium Flow"=0.0, "In Remote"=w243, "In Run"=w243, "In Bubbler"=w243, "In Active"=w243) -> ()  [unwired: 5 out]
                            }
                            frame True {
                              w246 = TRUE ("In Run")
                              n249 = property on="Run In" class="Bool (strict)"() -> ("Value"=w244:bool)  [unwired: 2 in, 2 out]
                              n250 = property on="In Flow" class="DigNum (strict)"() -> ("Value"=w245:dbl)  [unwired: 2 in, 2 out]
                              n251 = call "set_In.vi"("Indium Flow"=w245, "In Run"=w244, "In Bubbler"=w246, "In Active"=w246) -> ()  [unwired: 1 in, 5 out]
                            }
                          }
                        }
                        frame True {
                        }
                      }
                    }
                    frame #3 {
                      n252 = case shown="False" w247 {
                        frame False {
                          n253 = property on="PH3?" class="Bool (strict)"() -> ("Value"=w248:bool)  [unwired: 2 in, 2 out]
                          n254 = case shown="False" w248 {
                            frame False {
                              w249 = FALSE ("P_Gas Active")
                              n255 = call "set_P_gas.vi"("P_Gas Active"=w249, "P_Gas Flow"=0.0, "P_Gas In"=w249, "P_Gas H2 In"=w249, "P_Gas Run"=w249, "P_Gas Remote"=w249) -> ()  [unwired: 10 out]
                            }
                            frame True {
                              w253 = TRUE ("P_Gas Active")
                              n256 = property on="P Flow" class="DigNum (strict)"() -> ("Value"=w252:dbl)  [unwired: 2 in, 2 out]
                              n257 = property on="Run P" class="Bool (strict)"() -> ("Value"=w251:bool)  [unwired: 2 in, 2 out]
                              n258 = call "set_P_gas.vi"("P_Gas Active"=w253, "P_Gas Flow"=w252, "P_Gas In"=w253, "P_Gas Run"=w251) -> ()  [unwired: 2 in, 10 out]
                            }
                          }
                        }
                        frame True {
                        }
                      }
                    }
                    frame #4 {
                      n259 = case shown="False" w254 {
                        frame False {
                          n260 = property on="AsH3?" class="Bool (strict)"() -> ("Value"=w255:bool)  [unwired: 2 in, 2 out]
                          n261 = case shown="True" w255 {
                            frame False {
                              w256 = FALSE ("As_Gas Active")
                              n262 = call "set_As_gas.vi"("As_Gas Active"=w256, "As_Gas Flow"=0.0, "As_Gas In"=w256, "As_Gas H2"=w256, "As_Gas Run"=w256, "As_Gas Remote"=w256) -> ()  [unwired: 10 in]
                            }
                            frame True {
                              w259 = TRUE ("As_Gas Active")
                              n263 = property on="Run As" class="Bool (strict)"() -> ("Value"=w258:bool)  [unwired: 2 in, 2 out]
                              n264 = property on="AsH3 Flow" class="DigNum (strict)"() -> ("Value"=w260:dbl)  [unwired: 2 in, 2 out]
                              n265 = call "set_As_gas.vi"("As_Gas Active"=w259, "As_Gas Flow"=w260, "As_Gas In"=w259, "As_Gas Run"=w258) -> ()  [unwired: 12 in]
                            }
                          }
                        }
                        frame True {
                        }
                      }
                    }
                    frame #5 {
                      n266 = call "Set_Argument.vi"("Enable"=TRUE, "Argument"="run_started", "Argument List In"=w262) -> ("Argument List Out"=w261:string[])
                    }
                  }
                }
              }
            }
          }
        }
      }
    }
    frame "End" {
    }
    frame "Idle" {
    }
  }
  "Argument List Out" <- w10
